vi "SDCP Transfer Mode Request.vi"(1 "error in (no error)":errorcluster) -> (2 "BTR":bool, 3 "FTOR":bool, 4 "SFT":bool, 5 "error out":errorcluster)   [LabVIEW 2020]
uses:
  Typedefs/SDCP - Serial Port Control - Commands.ctl
  <vilib>/Instr/_visa.llb/VISA Flush IO Buffer Mask.ctl
panel:
  out "Number of iterations":i32
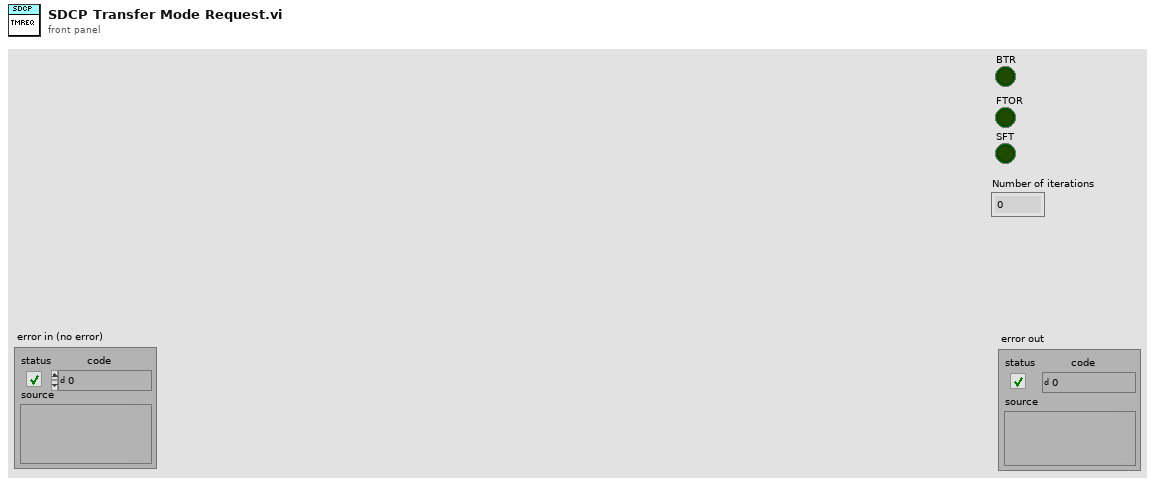
[diagram p1: front panel]
types:
  T1 = typedef "SDCP - Serial Port Control - Commands.ctl" = enum16{"Open", "Read", "Write", "Get instance", "Close"}
  T2 = typedef "VISA Flush IO Buffer Mask.ctl" = u16
  T3 = typedef "SDCP TMC Param.ctl" = cluster{"TMS_REQ":bool, "TMS_ACK":bool, "TMC_REQ":bool, "TMC_ACK":bool, "BTR_ENSTAT":bool, "FTOR_ENSTAT":bool, "SFT_ENSTAT":bool, "BTR_ENREQ":bool, "FTOR_ENREQ":bool, "SFT_ENREQ":bool, "MTR_ENREQ":bool, "MTR_ENACK":bool}
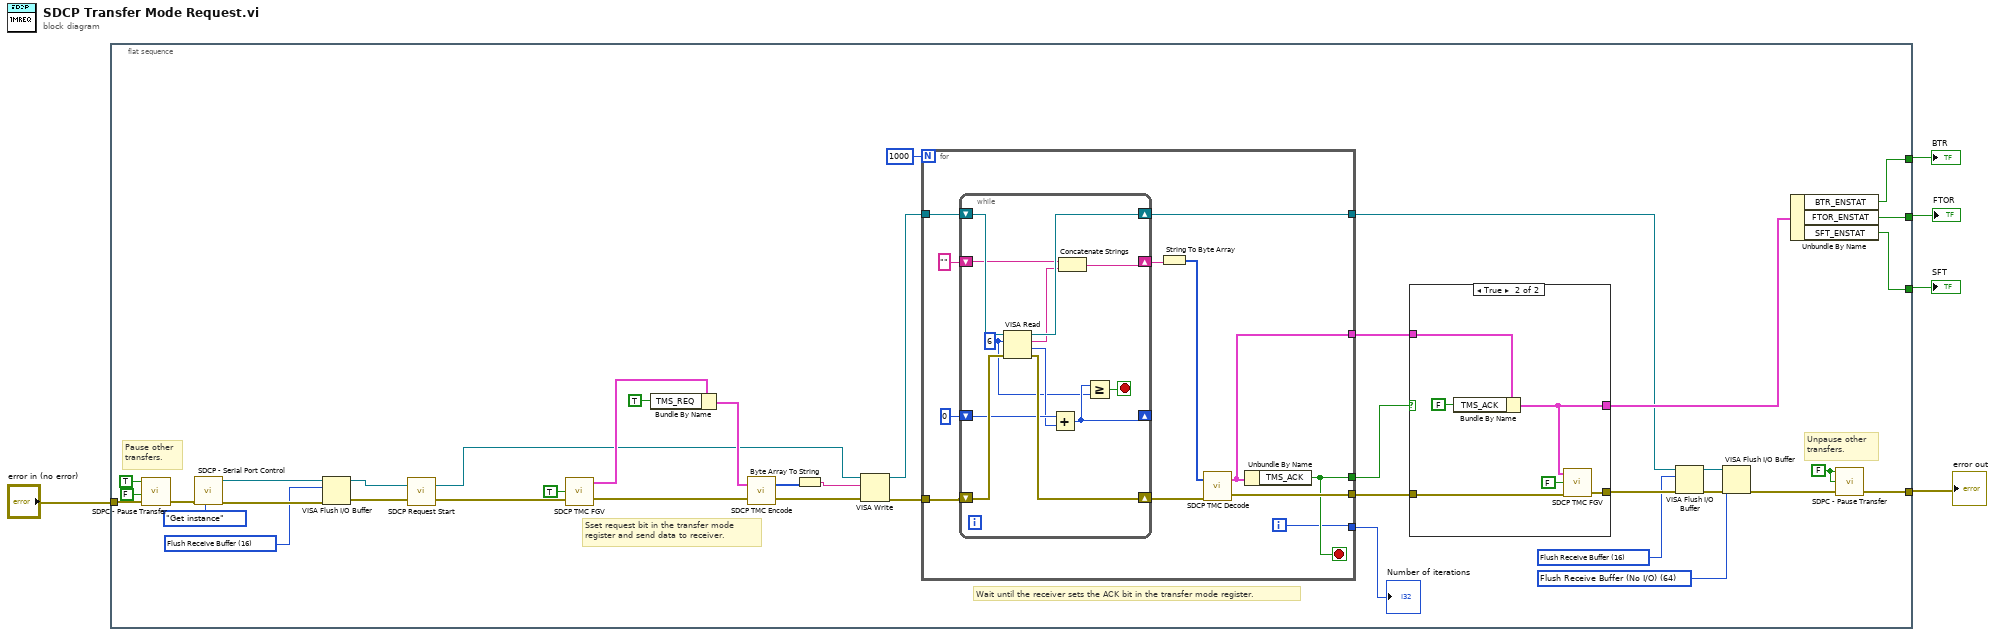
[diagram p0: block diagram]
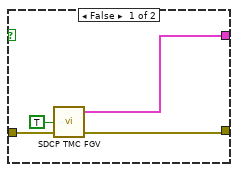
[diagram p2: hidden frame]
diagram:
  n1 = flat-sequence {
    tunnel: "error in (no error)" -> [w16]
    tunnel: [w12] -> w4
    tunnel: [w32] -> w3
    tunnel: [w31] -> w2
    tunnel: [w30] -> w1
    frame #0 {
      w6 = FALSE ("Pause transfer")
      w17 = T2 64 items=["Flush Receive Buffer"=16, "Write Transmit Buffer to Device"=32, "Flush Receive Buffer (No I/O)"=64, "Flush Transmit Buffer"=128] ("Mask")
      w20 = T2 16 items=["Flush Receive Buffer"=16, "Write Transmit Buffer to Device"=32, "Flush Receive Buffer (No I/O)"=64, "Flush Transmit Buffer"=128] ("Mask")
      w23 = T2 16 items=["Flush Receive Buffer"=16, "Write Transmit Buffer to Device"=32, "Flush Receive Buffer (No I/O)"=64, "Flush Transmit Buffer"=128] ("Mask")
      # "Unpause other\ntransfers."
      # "Pause other\ntransfers."
      # "Wait until the receiver sets the ACK bit in the transfer mode register."
      # "Sset request bit in the transfer mode \nregister and send data to receiver."
      n2 = call "SDPC - Pause Transfer.vi"("error in (no error)"=w16, "RD/nWR"=FALSE, "Pause transfer"=TRUE) -> ("error out"=w15:errorcluster)  [unwired: 1 in, 1 out]
      n3 = call "SDCP - Serial Port Control.vi"("Command"=SDCP_-_Serial_Port_Control_-_Commands."Get instance", "error in (no error)"=w15) -> ("error out"=w25:errorcluster, "VISA out"=w24:refnum<visa-resource-name>)  [unwired: 6 in, 2 out]
      n4 = VISA Flush I/O Buffer(VISA resource name=w24, mask (16)=w23, error in (no error)=w25) -> (VISA resource name out=w11:refnum<visa-resource-name>, error out=w10:errorcluster)
      n5 = call "SDCP Request Start.vi"("error in (no error)"=w10, "COM Port"=w11) -> ("error out"=w9:errorcluster, "COM Port Out"=w8:refnum<visa-resource-name>)
      n6 = call "SDCP TMC FGV.vi"("error in (no error)"=w9, "RD/nWR"=TRUE) -> ("error out"=w42:errorcluster, "TMC out"=w45:T3)  [unwired: 2 in]
      n7 = Bundle By Name(cluster=w45, "TMS_REQ"=TRUE) -> (w41:T3)
      n8 = call "SDCP TMC Encode.vi"("error in (no error)"=w42, "SDCP TMC Param"=w41) -> ("error out"=w40:errorcluster, "Encoded frame"=w38:u8[])
      n9 = Byte Array To String(unsigned byte array=w38) -> (string=w37:string)
      n10 = VISA Write(VISA resource name=w8, write buffer=w37, error in (no error)=w40) -> (VISA resource name out=w35:refnum<visa-resource-name>, error out=w36:errorcluster)  [unwired: 1 out]
      n11 = for {
        N: 1000 -> [_]
        tunnel: w36 -> [w67]
        tunnel: w35 -> [w66]
        tunnel: [w60] -> w33
        tunnel: [w59] -> w34
        tunnel: [w58] -> w27
        tunnel: [w57] -> w28
        tunnel: [w56] -> w21
        i -> [w57]
        stop <- w58 stop-if-true
        n12 = while {
          shift-right: [w78] -> w63
          shift-left: w67 -> [w79]
          shift-right: [w70] -> _
          shift-left: u32 0 -> [w75]
          shift-right: [w76] -> w56
          shift-left: w66 -> [w77]
          shift-right: [w71] -> w62
          shift-left: "" -> [w73]
          stop <- w69 stop-if-true
          w68 = u32 6 ("byte count")
          n13 = VISA Read(VISA resource name=w77, byte count=w68, error in (no error)=w79) -> (VISA resource name out=w76:refnum<visa-resource-name>, read buffer=w72:string, return count=w74:u32, error out=w78:errorcluster)
          n14 = Add(x=w75, y=w74) -> (x+y=w70:u32)
          n15 = Concatenate Strings(w73, w72) -> (w71:string)
          n16 = Greater Or Equal?(x=w70, y=w68) -> (x >= y?=w69:bool)
        }
        n17 = String To Byte Array(string=w62) -> (unsigned byte array=w61:u8[])
        n18 = call "SDCP TMC Decode.vi"("error in (no error)"=w63, "Frame"=w61) -> ("error out"=w59:errorcluster, "SDCP TMC out"=w60:T3)
        n19 = Unbundle By Name(w60) -> ("TMS_ACK"=w58:bool)
      }
      "Number of iterations" <- w28
      n20 = case shown="True" w27 {
        tunnel: w34 -> [w49 w55]
        tunnel: [w47 w53] -> w22
        tunnel: w33 -> [_ w51]
        tunnel: [w46 w50] -> w26
        frame False {
          n21 = call "SDCP TMC FGV.vi"("error in (no error)"=w49, "RD/nWR"=TRUE) -> ("error out"=w47:errorcluster, "TMC out"=w46:T3)  [unwired: 2 in]
        }
        frame True {
          n22 = Bundle By Name(cluster=w51, "TMS_ACK"=FALSE) -> (w50:T3)
          n23 = call "SDCP TMC FGV.vi"("error in (no error)"=w55, "RD/nWR"=FALSE, "TMC in"=w50) -> ("error out"=w53:errorcluster)  [unwired: 1 in, 1 out]
        }
      }
      n24 = VISA Flush I/O Buffer(VISA resource name=w21, mask (16)=w20, error in (no error)=w22) -> (VISA resource name out=w18:refnum<visa-resource-name>, error out=w19:errorcluster)
      n25 = VISA Flush I/O Buffer(VISA resource name=w18, mask (16)=w17, error in (no error)=w19) -> (error out=w13:errorcluster)  [unwired: 1 out]
      n26 = Unbundle By Name(w26) -> ("BTR_ENSTAT"=w32:bool, "FTOR_ENSTAT"=w31:bool, "SFT_ENSTAT"=w30:bool)
      n27 = call "SDPC - Pause Transfer.vi"("error in (no error)"=w13, "RD/nWR"=w6, "Pause transfer"=w6) -> ("error out"=w12:errorcluster)  [unwired: 1 in, 1 out]
    }
  }
  "error out" <- w4
  "BTR" <- w3
  "FTOR" <- w2
  "SFT" <- w1
